vi "CalcRate.vi"(8 "error in (no error)":errorcluster, 10 "Refresh(ms)":u32=100) -> (0 "error out":errorcluster, 1 "updated?":bool, 2 "Rate / Hz":dbl)   [LabVIEW 2017]
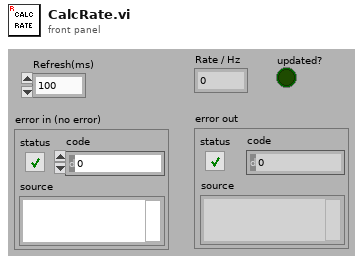
[diagram p1: front panel]
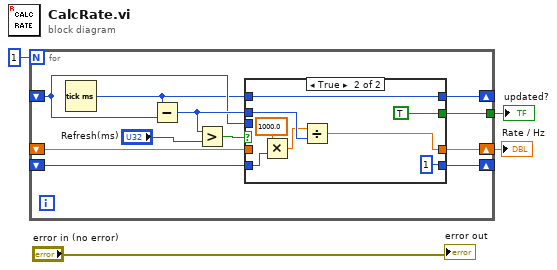
[diagram p0: block diagram]
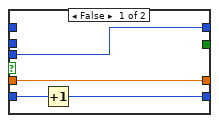
[diagram p2: hidden frame]
diagram:
  n1 = for {
    N: 1 -> [_]
    shift-right: [w12] -> _
    shift-left: _ -> [w9]
    shift-right: [w11] -> _
    shift-left: _ -> [w10]
    shift-right: [w8] -> w2
    shift-left: _ -> [w7]
    tunnel: [w5] -> w1
    n2 = Tick Count (ms)() -> (millisecond timer value=w6:u32)
    n3 = Subtract(x=w6, y=w9) -> (x-y=w13:u32)
    n4 = Greater?(x=w13, y="Refresh(ms)") -> (0:w14:bool)
    n5 = case shown="True" w14 {
      tunnel: w13 -> [_ w24]
      tunnel: [w18 1] -> w11
      tunnel: w10 -> [w19 w25]
      tunnel: w9 -> [w17 _]
      tunnel: [w17 w22] -> w12
      tunnel: w6 -> [_ w22]
      tunnel: [w16 w21] -> w8
      tunnel: w7 -> [w16 _]
      tunnel: [_ TRUE] -> w5
      frame False {
        n6 = Increment(x=w19) -> (x+1=w18:i32)
      }
      frame True {
        n7 = Multiply(x=1000.0, y=w25) -> (x*y=w23:dbl)
        n8 = Divide(x=w23, y=w24) -> (x/y=w21:dbl)
      }
    }
  }
  "Rate / Hz" <- w2
  "updated?" <- w1
  "error out" <- "error in (no error)"
